vi "CreateMotorPath.vi"(8 "Current Status":cluster{"Left?":bool, "Current Radius":dbl}, 11 "Planned Path":T2) -> (0 "New Commands?":bool, 3 "Motor Commands":T1(array[cluster]))   [LabVIEW 2011]
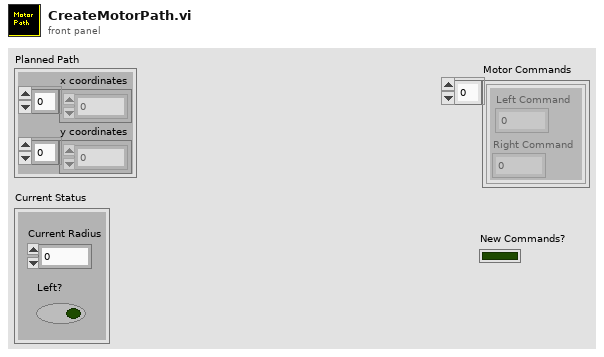
[diagram p1: front panel]
types:
  T1 = cluster{"Left Command":dbl, "Right Command":dbl}[]
  T2 = cluster{"x coordinates":i32[], "y coordinates":i32[]}
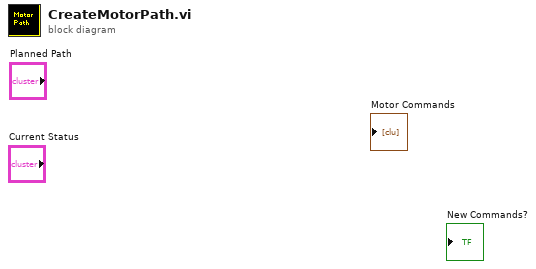
[diagram p0: block diagram]
diagram:
